vi "set array elements (dbl wfm arr).vi"(0 "array in":waveform(dbl)[](array[waveform]), 5 "start 1":i32, 7 "end 1":i32=-1, 9 "start 2":i32, 11 "end 2":i32=-1, 12 "val":dbl) -> (4 "array out":waveform(dbl)[](array[waveform]))   [LabVIEW 2012, in "common.lvlib"]
uses:
  common.lvlib
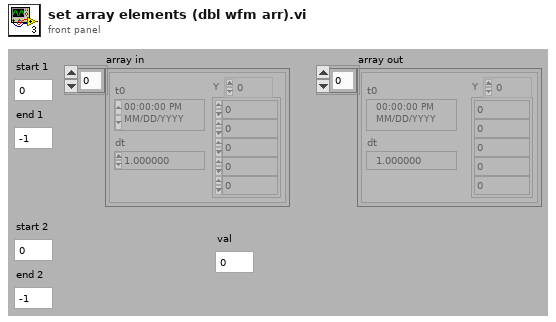
[diagram p1: front panel]
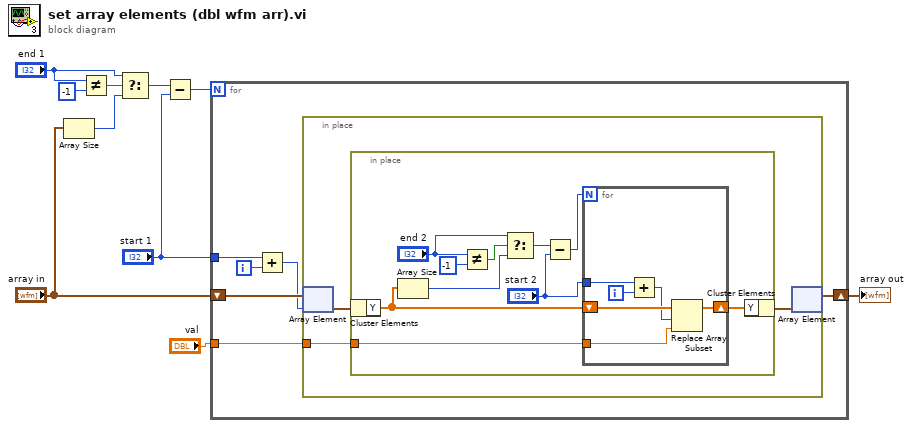
[diagram p0: block diagram]
diagram:
  n1 = Array Size(array="array in") -> (size(s)=w2:i32)
  n2 = Not Equal?(x="end 1", y=-1 ("x")) -> (x != y?=w7:bool)
  n3 = Select(t="end 1", s=w7, f=w2) -> (s? t:f=w4:i32)
  n4 = Subtract(x=w4, y="start 1") -> (x-y=w10:i32)
  n5 = for {
    N: w10 -> [_]
    shift-right: [w12] -> w8
    shift-left: "array in" -> [w14]
    tunnel: "val" -> [w11]
    tunnel: "start 1" -> [w15]
    i -> [w16]
    n6 = Add(x=w15, y=w16) -> (x+y=w13:i32)
    n7 = in-place {
      in-place-border: w11 -> [w17]
      n8 = in-place-array #1(w14, w13) -> (w19:waveform(dbl))
      n9 = in-place {
        in-place-border: w17 -> [w24]
        n10 = in-place-cluster #2(w19) -> ("Y"=w21:dbl[])
        n11 = Array Size(array=w21) -> (size(s)=w20:i32)
        n12 = Not Equal?(x="end 2", y=-1 ("x")) -> (x != y?=w27:bool)
        n13 = Select(t="end 2", s=w27, f=w20) -> (s? t:f=w25:i32)
        n14 = Subtract(x=w25, y="start 2") -> (x-y=w29:i32)
        n15 = for {
          N: w29 -> [_]
          tunnel: w24 -> [w32]
          shift-right: [w30] -> w22
          shift-left: w21 -> [w34]
          tunnel: "start 2" -> [w31]
          i -> [w35]
          n16 = Add(x=w31, y=w35) -> (x+y=w33:i32)
          n17 = Replace Array Subset(array=w34, new element=w32, index=w33) -> (w30:dbl[])
        }
        n18 = in-place-cluster #2("Y"=w22) -> (w18:waveform(dbl))
      }
      n19 = in-place-array #1(w18) -> (w12:waveform(dbl)[])  [unwired: 1 out]
    }
  }
  "array out" <- w8
